vi "Set Sparse Marker Indexes [SM] Core.vi"(8 "error in (no error)":errorcluster, 9 "Indexes Array":i64[](array[numeric]) caption="indexes array", 10 "Marker Name (\"\")":string caption="marker name (\"\")", 11 "IVI_Fgen in":refnum<class "IVI_Fgen.lvclass">) -> (0 "error out":errorcluster, 3 "IVI_Fgen out":refnum<class "IVI_Fgen.lvclass">)   [LabVIEW 2016, in "IVI_Fgen.lvlib" / "IVI_Fgen.lvclass"]
doc: "The VI sets the indexes associated with the sparse marker. These indexes may be coerced by the driver. Use the IviFgen Get Sparse Marker Indexes [SM] VI to find the coerced values.\n\nNote:\n\n(1) This VI is part of the IviFgenSparseMarker [SM] extension group."
uses:
  IVI_Fgen.lvclass
  IVI_Fgen.lvclass/IVI_Fgen.ctl
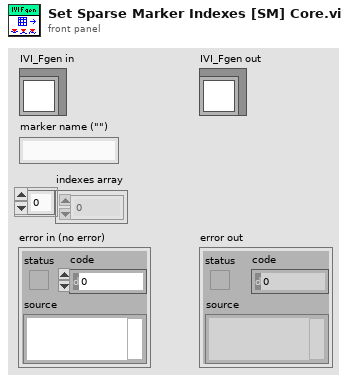
[diagram p1: front panel]
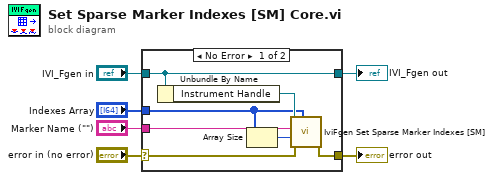
[diagram p0: block diagram]
diagram:
  n1 = case shown="No Error" "error in (no error)" {
    selector: "error in (no error)" -> [w11 w15]
    tunnel: [w10 w15] -> w5
    tunnel: [w13 w14] -> w3
    tunnel: "IVI_Fgen in" -> [w13 w14]
    tunnel: "Marker Name (\"\")" -> [w9 _]
    tunnel: "Indexes Array" -> [w8 _]
    frame No Error {
      n2 = Unbundle By Name(w13) -> ("Instrument Handle"=w12:refnum<k15>)
      n3 = Array Size(array=w8) -> (size(s)=w7:i32)
      n4 = call <vilib>:"IviFgen Set Sparse Marker Indexes [SM].vi"("Indexes Array"=w8, "error in (no error)"=w11, "Indexes Array Size"=w7, "Marker Name (\"\")"=w9, "instrument handle"=w12) -> ("error out"=w10:errorcluster)  [unwired: 5 in, 1 out]
    }
    frame Error {
    }
  }
  "error out" <- w5
  "IVI_Fgen out" <- w3
